vi "Get Template Page.vi"(7 "Target Name":string, 8 "error in (no error)":errorcluster, 10 "Item List":T1, 11 "Item Name":string) -> (0 "error out":errorcluster, 2 "Description":string, 3 "picture":picture, 5 "Found?":bool)   [LabVIEW 2021]
uses:
  Control/Item List.ctl
  Control/Item Info.ctl
  <vilib>/picture/picture.llb/imagedata.ctl
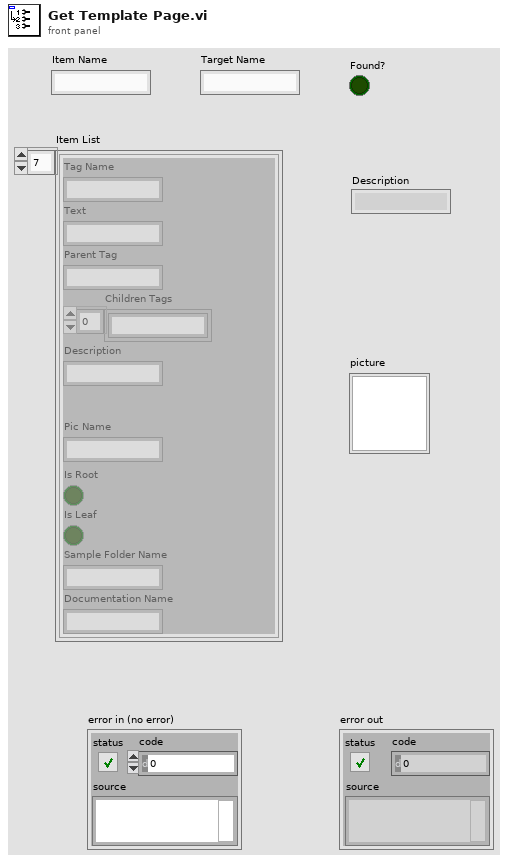
[diagram p1: front panel]
types:
  T1 = typedef "Item List.ctl" = T2[]
  T2 = typedef "Item Info.ctl" = cluster{"Tag Name":string, "Text":string, "Parent Tag":string, "Children Tags":string[], "Description":string, "Pic Name":string, "Is Root":bool, "Is Leaf":bool, "Sample Folder Name":string, "Documentation Name":string}
  T3 = typedef "imagedata.ctl" = cluster{"image type":i32, "image depth":i32, "image":u8[], "mask":u8[], "colors":u32[], "Rectangle":cluster{"left":i16, "top":i16, "right":i16, "bottom":i16}}
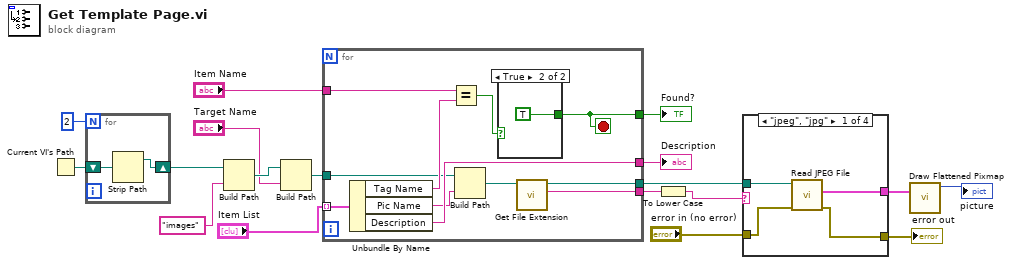
[diagram p0: block diagram]
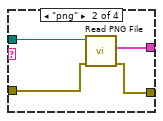
[diagram p2: hidden frame]
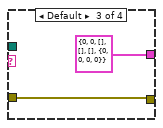
[diagram p3: hidden frame]
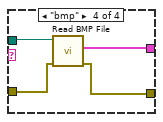
[diagram p4: hidden frame]
diagram:
  n1 = Current VI's Path() -> (path=w10:path)
  n2 = for {
    N: 2 -> [_]
    shift-right: [w19] -> w12
    shift-left: w10 -> [w20]
    n3 = Strip Path(path=w20) -> (stripped path=w19:path)  [unwired: 1 out]
  }
  n4 = Build Path(base path=w12, name or relative path="images") -> (appended path=w3:path)
  n5 = Build Path(base path=w3, name or relative path="Target Name") -> (appended path=w2:path)
  n6 = for {
    tunnel: "Item List" -> [w31] mode=indexing
    tunnel: "Item Name" -> [w29]
    tunnel: [w27] -> w15
    tunnel: [w26] -> w17
    tunnel: [w22] -> w9
    tunnel: w2 -> [w24]
    tunnel: [w21] -> w8
    stop <- w26 stop-if-true
    n7 = Unbundle By Name(w31) -> ("Tag Name"=w30:string, "Pic Name"=w25:string, "Description"=w27:string)
    n8 = Equal?(x=w29, y=w30) -> (x = y?=w28:bool)
    n9 = Build Path(base path=w24, name or relative path=w25) -> (appended path=w23:path)
    n10 = case shown="True" w28 {
      tunnel: [_ TRUE] -> w26
      frame False {
      }
      frame True {
      }
    }
    n11 = call <vilib>:"Get File Extension.vi"("file"=w23) -> ("lowercase file extension"=w21:string, "dup file"=w22:path)  [unwired: 6 in, 3 out]
  }
  "Found?" <- w17
  "Description" <- w15
  n12 = To Lower Case(string=w8) -> (all lower case string=w7:string)
  n13 = case shown="\"jpeg\", \"jpg\"" w7 {
    tunnel: w9 -> [w36 w40 _ w46]
    tunnel: [w35 w39 T3 {"image type"=0, "image depth"=0, "image"=[], "mask"=[], "colors"=[], "Rectangle"={"left"=0, "top"=0, "right"=0, "bottom"=0}} ("image data") w45] -> w6
    tunnel: "error in (no error)" -> [w34 w38 w41 w43]
    tunnel: [w33 w37 w41 w44] -> w4
    frame "jpeg", "jpg" {
      n14 = call <vilib>:"Read JPEG File.vi"("error in (no error)"=w34, "path to JPEG file"=w36) -> ("error out"=w33:errorcluster, "image data"=w35:T3)  [unwired: 7 in, 1 out]
    }
    frame "png" {
      n15 = call <vilib>:"Read PNG File.vi"("error in (no error)"=w38, "path to PNG file"=w40) -> ("error out"=w37:errorcluster, "image data"=w39:T3)  [unwired: 7 in, 1 out]
    }
    frame Default {
    }
    frame "bmp" {
      n16 = call <vilib>:"Read BMP File.vi"("error in (no error)"=w43, "path to BMP file"=w46) -> ("error out"=w44:errorcluster, "image data"=w45:T3)  [unwired: 7 in, 1 out]
    }
  }
  "error out" <- w4
  n17 = call <vilib>:"Draw Flattened Pixmap.vi"("image data"=w6) -> ("new picture"=→"picture":picture)  [unwired: 8 in]
